vi "SetFillLevel.vi"(0 "object in":refnum<class "CetoniPump.lvclass">, 2 "Flow":dbl, 3 "Level(ml)":dbl, 5 "error in (no error)":errorcluster) -> (14 "object out":refnum<class "CetoniPump.lvclass">, 19 "error out":errorcluster)   [LabVIEW 2024, in "CetoniPump.lvclass"]
uses:
  CetoniPump.lvclass
  CetoniPump.lvclass/CetoniPump.ctl
  Users/Lab user/AppData/Local/CETONI_SDK/lib/labview/labbCAN_Pump_API/labbCAN_Pump_API.lvlib
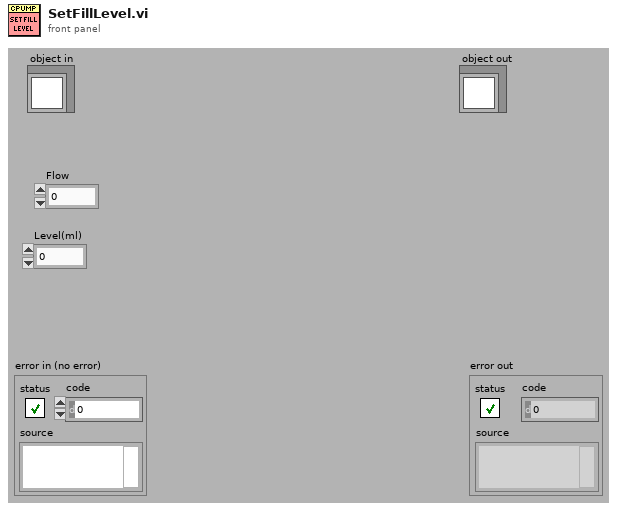
[diagram p1: front panel]
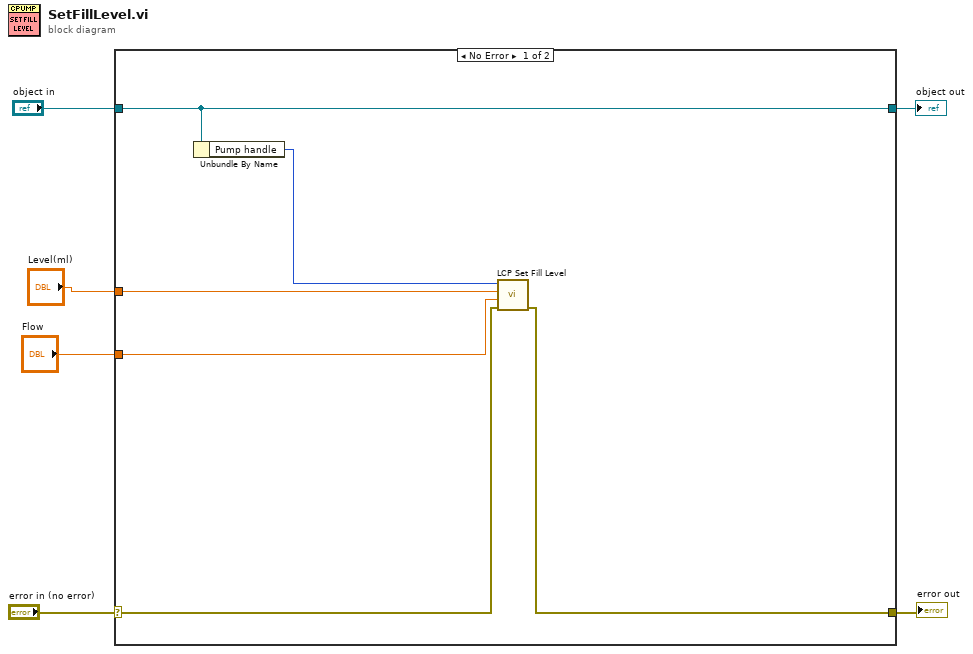
[diagram p0: block diagram]
diagram:
  n1 = case shown="No Error" "error in (no error)" {
    selector: "error in (no error)" -> [w8 w14]
    tunnel: [w7 w14] -> w5
    tunnel: [w12 w13] -> w3
    tunnel: "object in" -> [w12 w13]
    tunnel: "Level(ml)" -> [w10 _]
    tunnel: "Flow" -> [w9 _]
    frame No Error {
      n2 = Unbundle By Name(w12) -> ("Pump handle"=w11:i64)
      n3 = call "LCP Set Fill Level.vi"("error in (no error)"=w8, "Flow"=w9, "Level"=w10, "Pump Handle"=w11) -> ("error out"=w7:errorcluster)  [unwired: 7 in]
    }
    frame Error {
    }
  }
  "error out" <- w5
  "object out" <- w3
